vi "date_to_log_record_file_name.vi"(11 "Cluster":T1) -> (3 "st_logfilename":string)   [LabVIEW 2026]
doc: "Thids subVI creates the file name for log records"
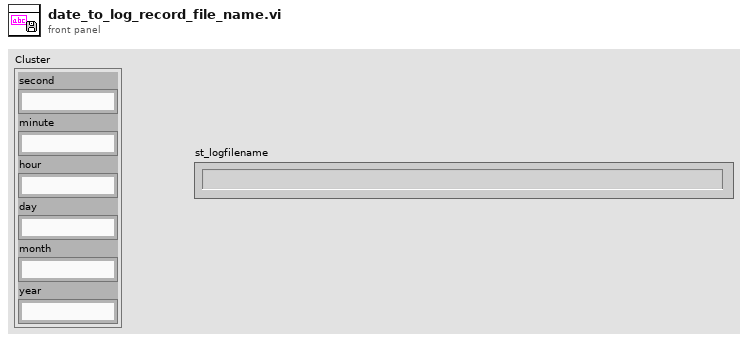
[diagram p1: front panel]
types:
  T1 = cluster{"second":string, "minute":string, "hour":string, "day":string, "month":string, "year":string}
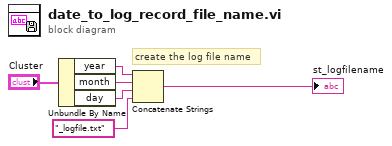
[diagram p0: block diagram]
diagram:
  # "create the log file name"
  n1 = Unbundle By Name("Cluster") -> ("year"=w4:string, "month"=w3:string, "day"=w2:string)
  n2 = Concatenate Strings(w4, w3, w2, "_logfile.txt") -> (→"st_logfilename":string)
